vi "Procura_no_Arquivo.vi"() -> (0 "Erro de Leitura=True":bool, 2 "Array":string[](array[string]))   [LabVIEW 2012]
uses:
  <vilib>/Utility/error.llb/whitespace.ctl
  Global_Telescopio.vi
  Shared_160.lvlib
panel:
  in  "Case Constant\n(See Context Help)":bool
  out "error out 3":errorcluster
  out "error out 2":errorcluster
  out "error out":errorcluster
  out "Ultima linha":string
  out "Saida":string
  out "dados lidos":string
  # "Temp     Hi    Low   Out    Dew  Wind  Wind   Wind    Hi    Hi   Wind   Heat    THW   THSW          Solar   Solar Hi Solar   UV    UV    Hi     Heat    Cool    In     In    In     In           Wind  Wind    ISS   Arc.\n  Date    Time     Out   Temp   Temp   Hum    Pt. Speed   Dir    Run Speed   Dir  Chill  Index  Index  Index   Bar     Rad.  Energy    Rad.  Index  Dose   UV     D-D     D-D    Temp   Hum    Dew   Heat     ET   Samp   Tx   Recept  Int."
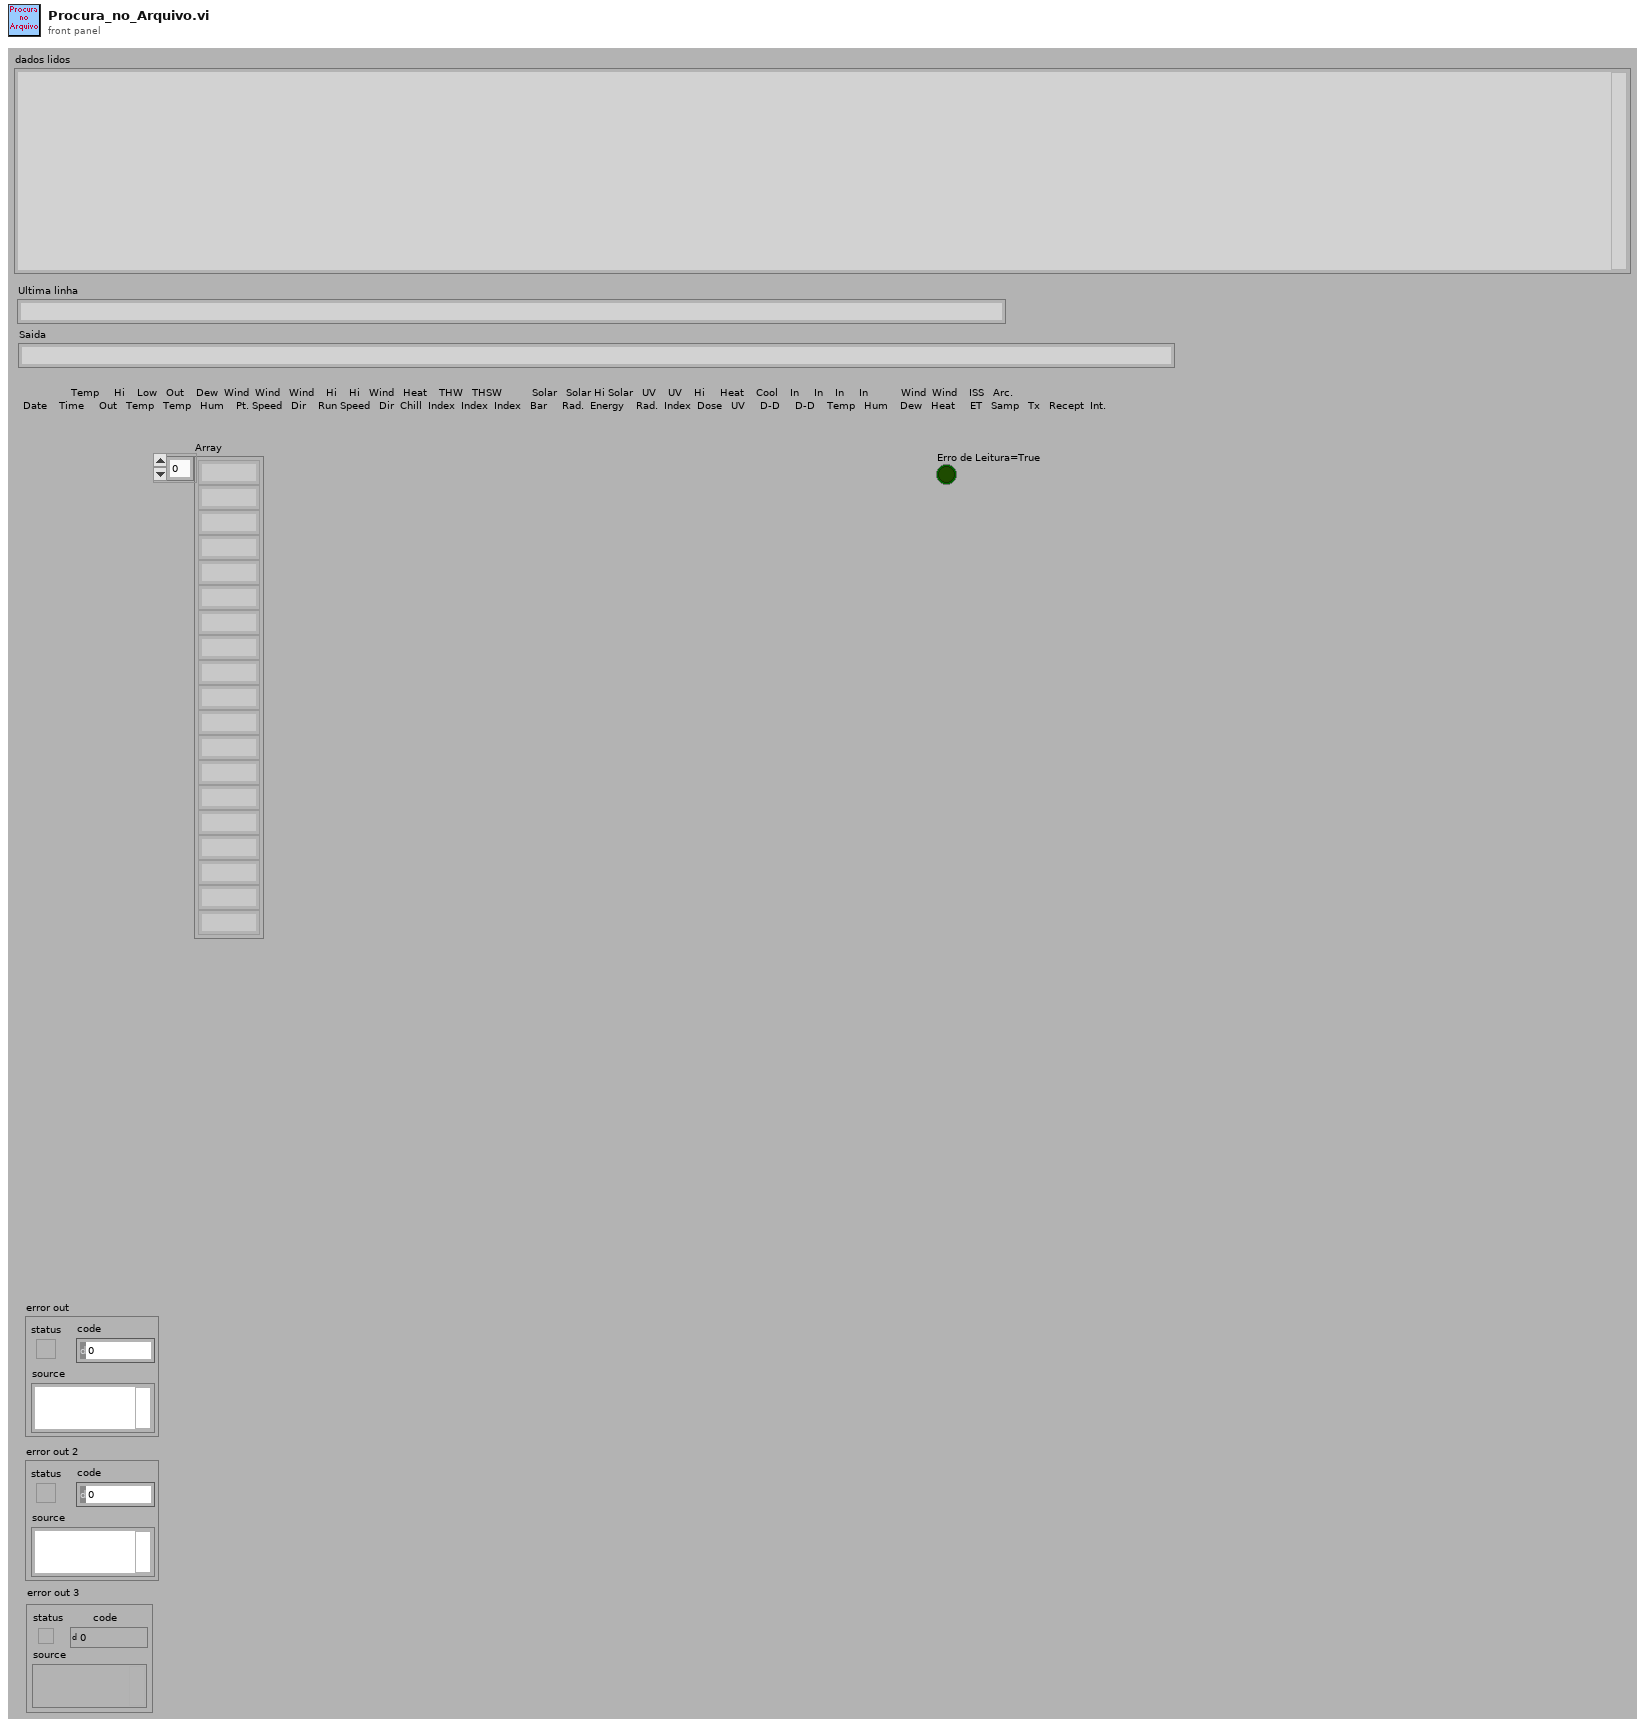
[diagram p1: front panel]
types:
  T1 = typedef "whitespace.ctl" = u16
  T2 = enum16{"open", "open or create", "create or replace", "create"}
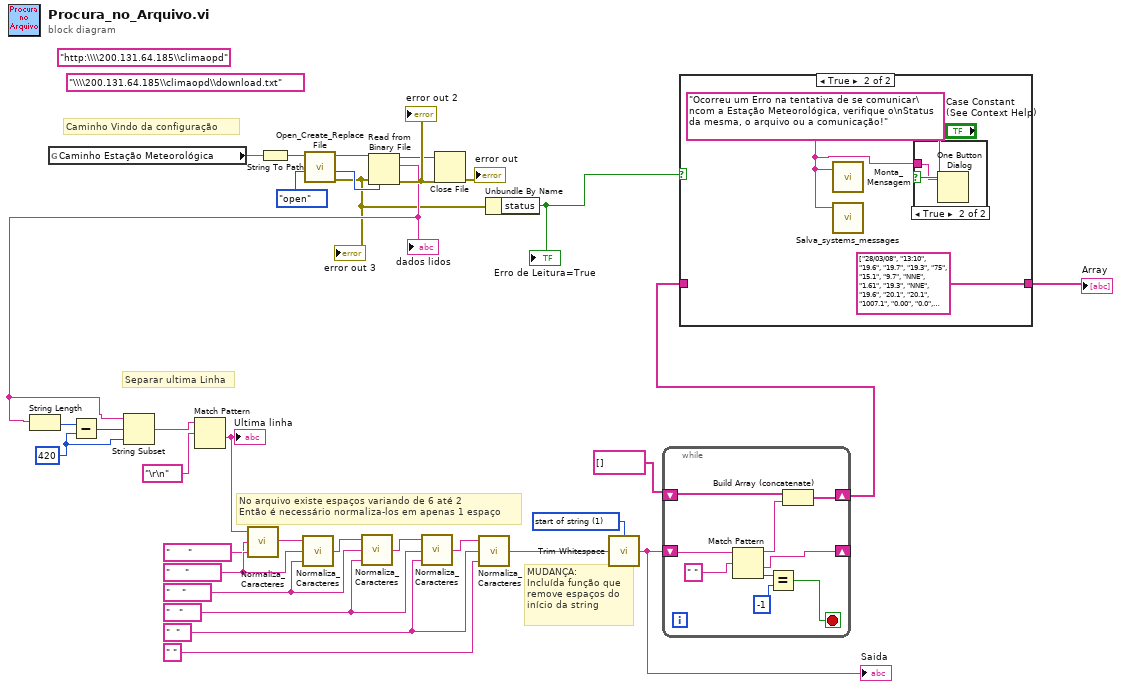
[diagram p0: block diagram]
diagram:
  w5 = T1 1 items=["both", "start of string", "end of string"] ("location (both)")
  w14 = 420 ("y")
  (unwired) "http:\\\\200.131.64.185\\climaopd"
  (unwired) "\\\\200.131.64.185\\climaopd\\download.txt" ("caminho final")
  w21 = "     "
  w25 = "  "
  w22 = "    "
  w26 = "   "
  # "MUDANÇA:\nIncluída função que\nremove espaços do\ninício da string"
  # "Caminho Vindo da configuração"
  # "Separar ultima Linha"
  # "No arquivo existe espaços variando de 6 até 2\nEntão é necessário normaliza-los em apenas 1 espaço"
  n1 = global read "Global_Telescopio.vi" "Caminho Estação Meteorológica"() -> (w9:string)
  n2 = String To Path(string=w9) -> (path=w17:path)
  n3 = call <vilib>:"Open_Create_Replace File.vi"("function (open:0)"=T2."open", "file path"=w17) -> ("error out"=w8:errorcluster, "file size (bytes)"=w32:i32, "refnum"=w29:refnum<file>)  [unwired: 6 in, 1 out]
  "error out 3" <- w8
  n4 = Read from Binary File(8:w8, 10:w32, 11:w29) -> (0:w31:errorcluster, 2:w13:string, 3:w30:refnum<file>)  [unwired: 3 in, 1 out]
  "dados lidos" <- w13
  "error out 2" <- w31
  n5 = String Length(string=w13) -> (length=w16:i32)
  n6 = Subtract(x=w16, y=w14) -> (x-y=w15:i32)
  n7 = String Subset(string=w13, offset (0)=w15, length (rest)=w14) -> (substring=w12:string)
  n8 = Match Pattern(string=w12, regular expression="\r\n") -> (after substring=w10:string)  [unwired: 1 in, 3 out]
  "Ultima linha" <- w10
  n9 = call "Normaliza_Caracteres.vi"("Trocar por:"=w21, "Procurar"="      ", "Entrada"=w10) -> ("Saida"=w19:string)  [unwired: 2 in]
  n10 = call "Normaliza_Caracteres.vi"("Trocar por:"=w22, "Procurar"=w21, "Entrada"=w19) -> ("Saida"=w23:string)  [unwired: 2 in]
  n11 = call "Normaliza_Caracteres.vi"("Trocar por:"=w26, "Procurar"=w22, "Entrada"=w23) -> ("Saida"=w28:string)  [unwired: 2 in]
  n12 = call "Normaliza_Caracteres.vi"("Trocar por:"=w25, "Procurar"=w26, "Entrada"=w28) -> ("Saida"=w27:string)  [unwired: 2 in]
  n13 = Close File(refnum=w30, error in=w31) -> (error out=→"error out":errorcluster)  [unwired: 1 out]
  n14 = call "Normaliza_Caracteres.vi"("Trocar por:"=" ", "Procurar"=w25, "Entrada"=w27) -> ("Saida"=w6:string)  [unwired: 2 in]
  n15 = Unbundle By Name(w8) -> ("status"=w4:bool)
  "Erro de Leitura=True" <- w4
  n16 = call <vilib>:"Trim Whitespace.vi"("string"=w6, "location (both)"=w5) -> ("trimmed string"=w7:string)
  "Saida" <- w7
  n17 = while {
    shift-right: [w36] -> _
    shift-left: w7 -> [w37]
    shift-right: [w35] -> w3
    shift-left: string[] [] -> [w34]
    stop <- w38 stop-if-true
    n18 = Match Pattern(string=w37, regular expression=" ") -> (before substring=w42:string, after substring=w36:string, offset past match=w40:i32)  [unwired: 1 in, 1 out]
    n19 = Equal?(x=w40, y=-1) -> (x = y?=w38:bool)
    n20 = Build Array (concatenate)(w34, w42) -> (w35:string[])
  }
  n21 = case shown="True" w4 {
    tunnel: w3 -> [w43 _]
    tunnel: [w43 string[] ["28/03/08", "13:10", "19.6", "19.7", "19.3", "75", "15.1", "9.7", "NNE", "1.61", "19.3", "NNE", "19.6", "20.1", "20.1", "1007.1", "0.00", "0.0", "0.000", "0.009", "24.7", "45", "12.0", "24.4", "25.6", "---", "49", "---", "228", "1", "100.0", "10", "\r\n", "", "", "", "", ""] ("Array 2")] -> w2
    frame False {
    }
    frame True {
      w44 = "Ocorreu um Erro na tentativa de se comunicar\ncom a Estação Meteorológica, verifique o\nStatus da mesma, o arquivo ou a comunicação!" ("message")
      n22 = call "Monta_Mensagem.vi"("Mensagem"=w44) -> ()  [unwired: 2 in]
      n23 = call "Salva_systems_messages.vi"("Mensagem"=w44) -> ()  [unwired: 5 in]
      n24 = case shown="True" "Case Constant\n(See Context Help)" {
        tunnel: w44 -> [_ w47]
        frame False {
        }
        frame True {
          n25 = One Button Dialog(message=w47) -> ()  [unwired: 1 in, 1 out]
        }
      }
    }
  }
  "Array" <- w2
